vi "Read Pulse Recorder Configuration.vi"(8 "error in (no error)":errorcluster, 11 "RP I-V in":refnum<class "RP I-V.lvclass">) -> (0 "error out":errorcluster, 2 "Configuration":T1={"Pre-trigger duration"=0.01, "Post-trigger duration"=0.1, "Rate"=1000000.0, "Ranges"=[10.0], "Re-name channels"=[], "Active channels"="0:1", "External clock"=FALSE} {"Rate" format="%#_8pHz"; "Post-trigger duration" format="%#_6ps"; "Pre-trigger duration" format="%#_6ps"; "Ranges" format="%#_6pV"}, 3 "RP I-V out":refnum<class "RP I-V.lvclass">)   [LabVIEW 2018, in "RP I-V.lvclass"]
uses:
  RP I-V.lvclass
  NHMFL_Core/Libraries/Instruments/Pulse Driver/Pusle Driver Configuration.ctl
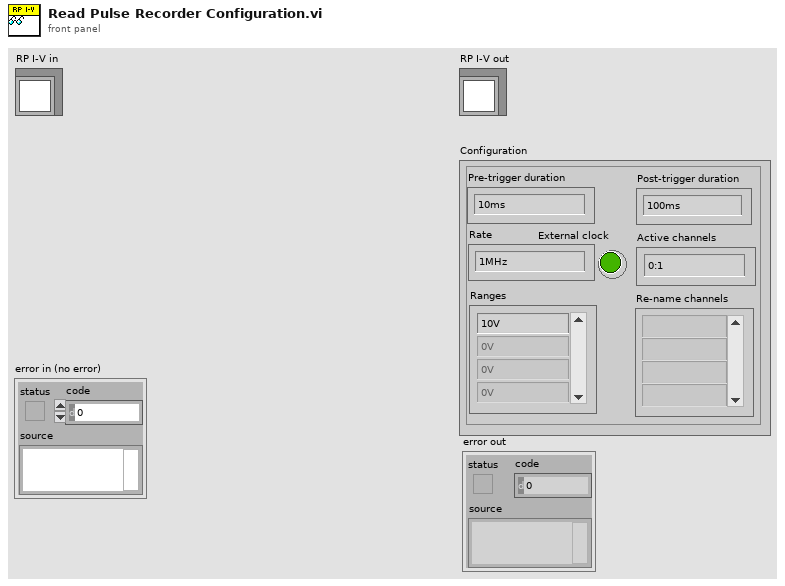
[diagram p1: front panel]
types:
  T1 = typedef "Pusle Driver Configuration.ctl" = cluster{"Pre-trigger duration":dbl, "Post-trigger duration":dbl, "Rate":dbl, "Ranges":dbl[], "Re-name channels":string[], "Active channels":string, "External clock":bool}
  T2 = typedef "RP I-V Configuration.ctl" = cluster{"I-V parameters":T3, "Ranges":dbl[], "Pre-trigger duration":dbl, "Post-trigger duration":dbl, "Output delay":dbl}
  T3 = typedef "I-V parameters.ctl" = cluster{"Start magnitude":dbl, "Magnitude increment":dbl, "End magnitude":dbl, "Ramp length":i32, "Top  length":i32, "Threshold ":dbl, "Processing delay":u16, "Valhalla range":dbl, "Interpolation":i32, "Stop after":u16, "Detector window":i32}
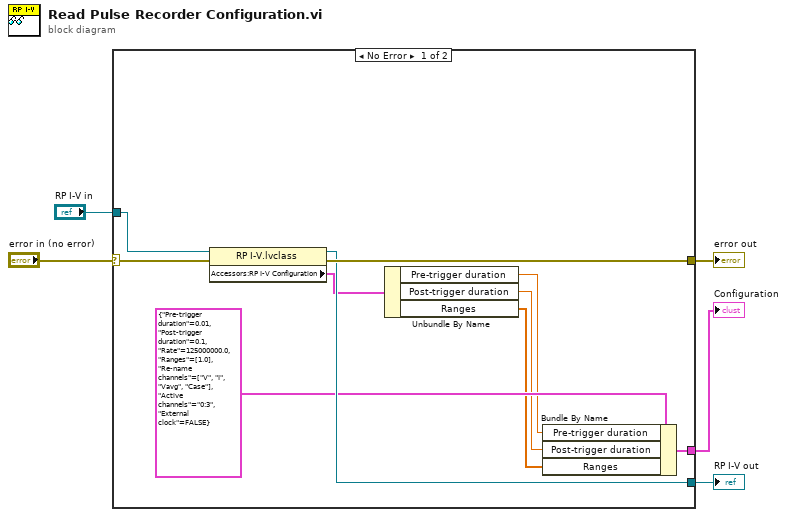
[diagram p0: block diagram]
diagram:
  n1 = case shown="No Error" "error in (no error)" {
    selector: "error in (no error)" -> [w14 w16]
    tunnel: [w13 w16] -> w3
    tunnel: [w12 w17] -> w1
    tunnel: "RP I-V in" -> [w15 w17]
    tunnel: [w10 _] -> w2
    frame No Error {
      n2 = property class="RP I-V.lvclass"(reference=w15, error in=w14) -> (reference out=w12:refnum<class "RP I-V.lvclass">, error out=w13:errorcluster, "Accessors:RP I-V Configuration"=w6:T2)
      n3 = Unbundle By Name(w6) -> ("Pre-trigger duration"=w9:dbl, "Post-trigger duration"=w8:dbl, "Ranges"=w7:dbl[])
      n4 = Bundle By Name(cluster=T1 {"Pre-trigger duration"=0.01, "Post-trigger duration"=0.1, "Rate"=125000000.0, "Ranges"=[1.0], "Re-name channels"=["V", "I", "Vavg", "Case"], "Active channels"="0:3", "External clock"=FALSE} ("Configuration"), "Pre-trigger duration"=w9, "Post-trigger duration"=w8, "Ranges"=w7) -> (w10:T1)
    }
    frame Error {
    }
  }
  "error out" <- w3
  "RP I-V out" <- w1
  "Configuration" <- w2
